vi "sequencerCWTopLevel.vi"() -> ()   [LabVIEW 2014]
uses:
  Controls/measVoltState.ctl
  sequencerState.ctl
  Controls/SPstate.ctl
  Controls/heinzingerSelect.ctl
  Controls/triggerTypes.ctl
  Controls/selectTrigger.ctl
  Controls/triggerEdge.ctl
  OutBits/OutbitsStateControl.ctl
  <vilib>/rvi/Emulation/niFpgaGetClockAttributes.vi
  <vilib>/rvi/Emulation/niFpgaSctlEmulationGetInTimedLoop.vi
  <vilib>/rvi/Emulation/niFpgaEmulationReportErrorSimple.vi
  Trigger/triggerGlobalVars.vi
  <vilib>/rvi/Emulation/niFpgaProcessEmulError.vi
  ScanTrigger/scanTriggerGlobalVars.vi
  StepTrigger/stepTriggerGlobalVars.vi
  sequencerGlobVars.vi
  MeasVolt/measVoltGlobVars.vi
  QueueHandler/queueHandlerGlobals.vi
  SimpleCounter/SCGlobVars.vi
  HeinzingerControl/heinzingerControlGlobals.vi
  OutBits/OutbitsGlobalVars.vi
  ScanDeviceLogic/scanDeviceGlobalVars.vi
  <vilib>/rvi/Emulation/niFpgaCriticalErrorInLSC.vi
panel:
  out "internalDacAvailable":bool
  in  "ScanDevice":enum16{"internal DAC", "external Python"}(ring)
  in  "scanDevSet":bool
  in  "scanDevTimeout(10ns)":i32
  in  "stepTrigDelay10ns":u32
  in  "softwareStepTrigger":bool
  in  "stepTriggerEdge":T1=enum."true-false"
  in  "stepTriggerTypes":T2
  in  "selectStepTrigger":T3
  in  "softwareScanTrigger":bool
  in  "scanTriggerEdge":T1=enum."true-false"
  in  "scanTrigDelay10ns":u32
  in  "selectScanTrigger":T3
  in  "scanTriggerTypes":T2
  out "nOfCmdsOutbit2":u32
  out "nOfCmdsOutbit1":u32
  out "nOfCmdsOutbit0":u32
  out "OutBitsState":T4
  in  "softwareTrigger":bool
  in  "pause":bool
  in  "stopVoltMeas":bool caption="measVoltStop"
  in  "measVoltCompleteDest":T5(ring)
  in  "dac0VRegister":u32=1572792 format="%024b"
  in  "triggerEdge":T1=enum."true-false"
  in  "trigDelay10ns":u32
  in  "selectTrigger":T3
  in  "triggerTypes":T2
  out "postAccOffsetVoltState":T6
  in  "postAccOffsetVoltControl":T6=enum."loading"
  out "SPerrorCount":u8
  out "SPstate":T7
  in  "dwellTime10ns":u32=2000000
  out "SPCtrQuWriteTimeout":bool
  in  "VoltOrScaler?":bool
  in  "dacStepSize20Bit":i32
  in  "dacStartRegister20Bit":i32
  in  "nOfSteps":i32
  in  "nOfScans":i32
  in  "invertScan":bool
  in  "waitForKepco(us)":u32
  in  "waitAfterReset(us)":u32 caption="waitForDmm(25nsTicks)"
  in  "measVoltPulseLength(25ns)":i32
  in  "measVoltTimeout(10ns)":i32 caption="measVoltTimeout(25ns)"
  in  "timedOutWhileHandshake":bool
  out "seqState":T8
  in  "cmdByHost":T8
  in  "abort":bool
  in  "halt":bool
  in  "hostConfirmsHzOffsetIsSet":bool
  out "measVoltState":T9
  out "DACQuWriteTimeout":bool
  # "Step Trigger"
  # "Step Trigger"
  # "Scan Trigger"
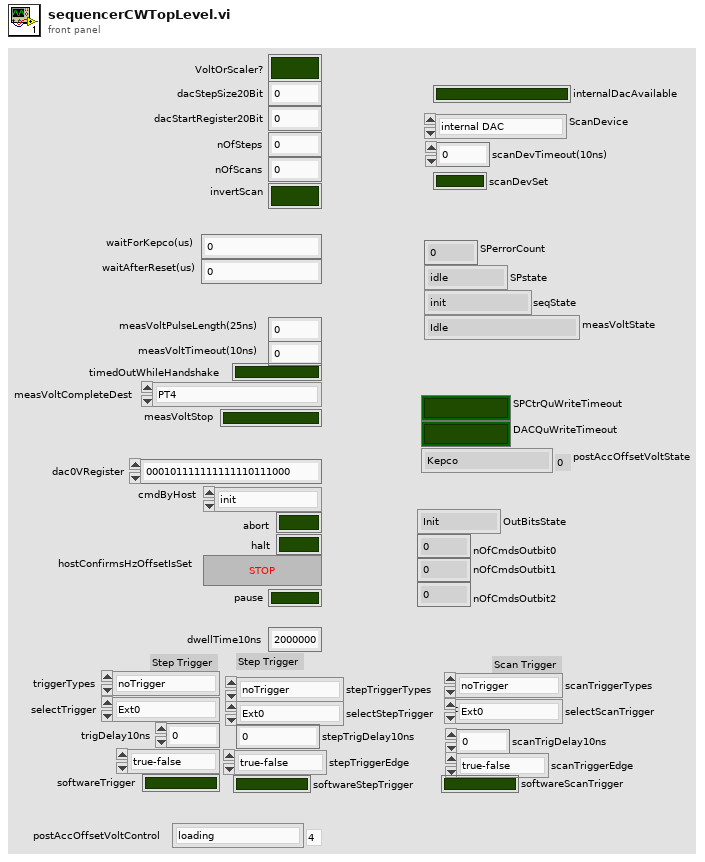
[diagram p1: front panel]
types:
  T1 = typedef "triggerEdge.ctl" = enum8{"either", "false-true", "true-false"}
  T2 = typedef "triggerTypes.ctl" = enum16{"noTrigger", "singleHitDelay", "singleHit", "software", "sweep"}
  T3 = typedef "selectTrigger.ctl" = enum8{"Ext0", "Ext1", "Ext2", "Ext3", "Ext4", "Ext5", "Ext6", "Ext7", "Int0", "Int1", "Int2", "Int3", "Int4", "Int5", "Int6", "Int7"}
  T4 = typedef "OutbitsStateControl.ctl" = enum16{"Init", "Idle", "loading", "listening", "clearing", "error"}
  T5 = enum16{"PT4", "C1D30", "C1D31", "PT4_C1D30", "PT4_C1D31", "PT4_C1D30_C1D31", "C1D30_C1D31"}
  T6 = typedef "heinzingerSelect.ctl" = enum8{"Kepco", "Heinzinger0", "Heinzinger1", "Heinzinger2", "loading"}
  T7 = typedef "SPstate.ctl" = enum16{"idle", "scanning", "done", "error"}
  T8 = typedef "sequencerState.ctl" = enum16{"init", "idle", "measureOffset", "measureTrack", "measComplete", "error"}
  T9 = typedef "measVoltState.ctl" = enum16{"Idle", "sendMeasRequest", "waitUntilDone", "done"}
  T10 = cluster{"SCLK":refnum<k21>, "CS":refnum<k21>, "MOSI":refnum<k21>, "MISO":refnum<k21>}
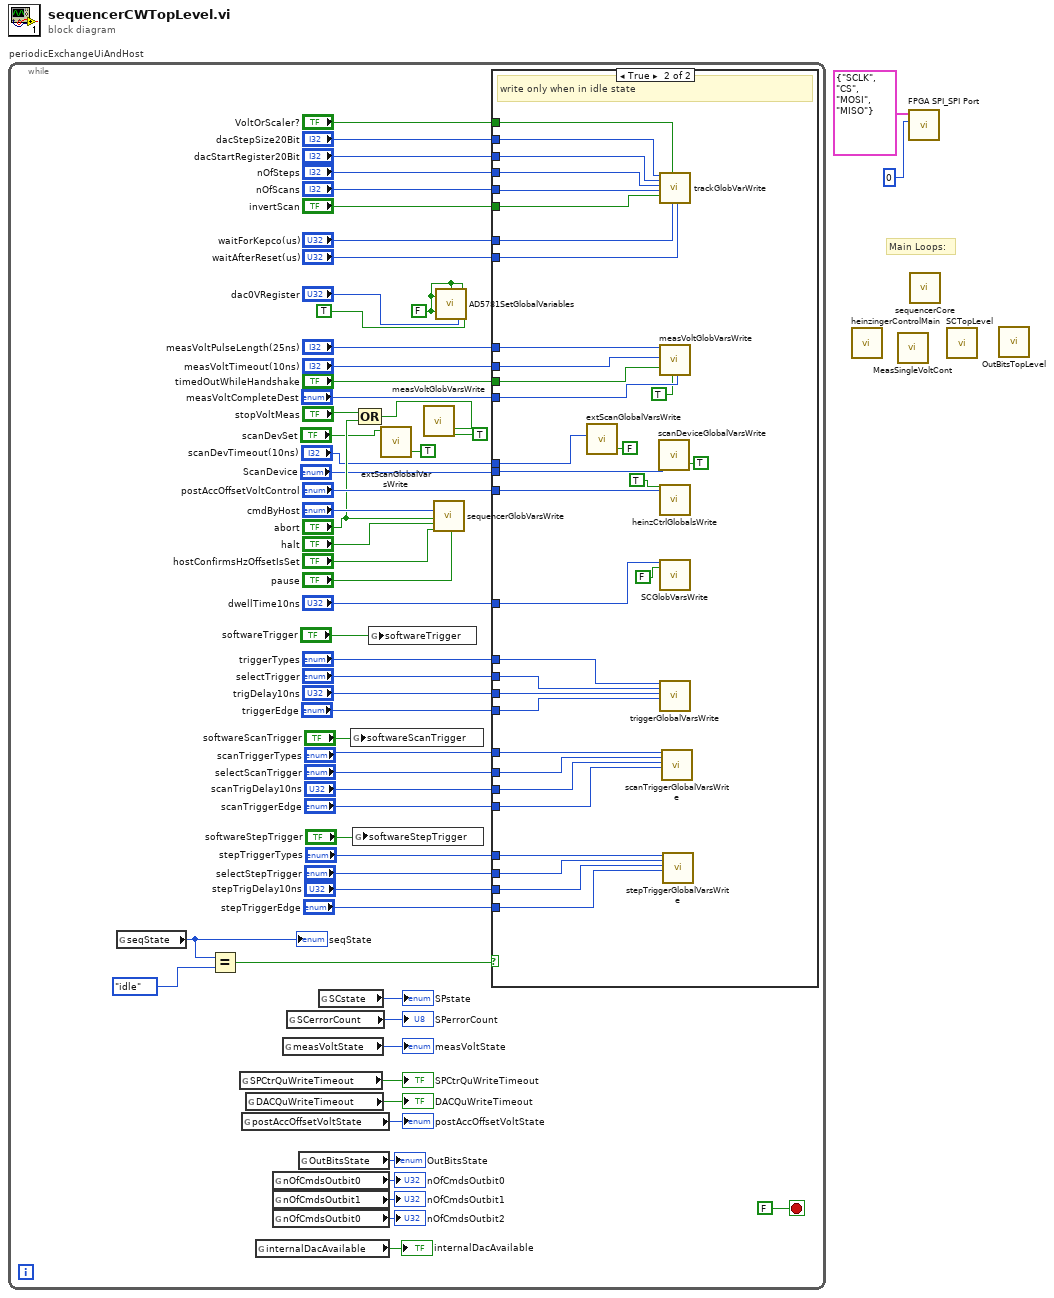
[diagram p0: block diagram]
diagram:
  # "Main Loops:"
  n1 = while "periodicExchangeUiAndHost" {
    stop <- FALSE stop-if-true
    w31 = FALSE ("write setDACRegister")
    n2 = global read "sequencerGlobVars.vi" "seqState"() -> (w43:T8)
    "seqState" <- w43
    n3 = Equal?(x=w43, y=sequencerState."idle") -> (x = y?=w60:bool)
    n4 = global read "queueHandlerGlobals.vi" "SPCtrQuWriteTimeout"() -> (→"SPCtrQuWriteTimeout":bool)
    n5 = global read "heinzingerControlGlobals.vi" "postAccOffsetVoltState"() -> (→"postAccOffsetVoltState":T6)
    n6 = global read "queueHandlerGlobals.vi" "DACQuWriteTimeout"() -> (→"DACQuWriteTimeout":bool)
    n7 = global read "scanDeviceGlobalVars.vi" "internalDacAvailable"() -> (→"internalDacAvailable":bool)
    n8 = global read "OutbitsGlobalVars.vi" "nOfCmdsOutbit0"() -> (→"nOfCmdsOutbit0":u32)
    n9 = global read "OutbitsGlobalVars.vi" "nOfCmdsOutbit1"() -> (→"nOfCmdsOutbit1":u32)
    n10 = global read "OutbitsGlobalVars.vi" "nOfCmdsOutbit0"() -> (→"nOfCmdsOutbit2":u32)
    n11 = global read "measVoltGlobVars.vi" "measVoltState"() -> (→"measVoltState":T9)
    n12 = global read "SCGlobVars.vi" "SCerrorCount"() -> (→"SPerrorCount":u8)
    n13 = global read "OutbitsGlobalVars.vi" "OutBitsState"() -> (→"OutBitsState":T4)
    n14 = global read "SCGlobVars.vi" "SCstate"() -> (→"SPstate":T7)
    n15 = global write "scanTriggerGlobalVars.vi" "softwareScanTrigger"("softwareScanTrigger") -> ()
    n16 = global write "stepTriggerGlobalVars.vi" "softwareStepTrigger"("softwareStepTrigger") -> ()
    n17 = Compound Arithmetic op=OR("stopVoltMeas", "abort") -> (w25:bool)
    n18 = global write "triggerGlobalVars.vi" "softwareTrigger"("softwareTrigger") -> ()
    n19 = call "extScanGlobalVarsWrite.vi"("WriteDevSet"=TRUE, "scanDevSet"="scanDevSet") -> ()  [unwired: 10 in]
    n20 = call "measVoltGlobVarsWrite.vi"("stopVoltMeas"=w25, "writeStopVoltMeas"=TRUE) -> ()  [unwired: 18 in]
    n21 = call "sequencerGlobVarsWrite.vi"("cmdByHost"="cmdByHost", "abort"="abort", "halt"="halt", "hostConfirmsHzOffsetIsSet"="hostConfirmsHzOffsetIsSet", "pause"="pause") -> ()  [unwired: 15 in]
    n22 = call "AD5781SetGlobalVariables.vi"("write actDACRegister"=w31, "write setDACRegister"=w31, "write DacStateCmdByHost"=w31, "dac0VRegister"="dac0VRegister", "writeSpiGlobals"=w31, "write dac0VRegister"=TRUE) -> ()  [unwired: 14 in]
    n23 = case shown="True" w60 {
      tunnel: "VoltOrScaler?" -> [_ w94]
      tunnel: "dacStepSize20Bit" -> [_ w93]
      tunnel: "dacStartRegister20Bit" -> [_ w92]
      tunnel: "nOfSteps" -> [_ w91]
      tunnel: "nOfScans" -> [_ w90]
      tunnel: "invertScan" -> [_ w89]
      tunnel: "waitForKepco(us)" -> [_ w88]
      tunnel: "waitAfterReset(us)" -> [_ w87]
      tunnel: "measVoltPulseLength(25ns)" -> [_ w86]
      tunnel: "measVoltTimeout(10ns)" -> [_ w85]
      tunnel: "timedOutWhileHandshake" -> [_ w84]
      tunnel: "dwellTime10ns" -> [_ w82]
      tunnel: "postAccOffsetVoltControl" -> [_ w80]
      tunnel: "triggerTypes" -> [_ w79]
      tunnel: "selectTrigger" -> [_ w78]
      tunnel: "trigDelay10ns" -> [_ w77]
      tunnel: "triggerEdge" -> [_ w76]
      tunnel: "measVoltCompleteDest" -> [_ w75]
      tunnel: "scanTriggerTypes" -> [_ w73]
      tunnel: "selectScanTrigger" -> [_ w72]
      tunnel: "scanTrigDelay10ns" -> [_ w71]
      tunnel: "scanTriggerEdge" -> [_ w70]
      tunnel: "stepTriggerTypes" -> [_ w69]
      tunnel: "selectStepTrigger" -> [_ w68]
      tunnel: "stepTrigDelay10ns" -> [_ w67]
      tunnel: "stepTriggerEdge" -> [_ w66]
      tunnel: "ScanDevice" -> [_ w65]
      tunnel: "scanDevTimeout(10ns)" -> [_ w64]
      frame False {
      }
      frame True {
        # "write only when in idle state"
        n24 = call "extScanGlobalVarsWrite.vi"("WriteDevSet"=FALSE, "scanDevTimeout(10ns)"=w64) -> ()  [unwired: 10 in]
        n25 = call "scanDeviceGlobalVarsWrite.vi"("ChooseScanDevice"=TRUE, "ScanDevice"=w65) -> ()  [unwired: 10 in]
        n26 = call "trackGlobVarWrite.vi"("dacStepSize20Bit"=w93, "dacStartRegister20Bit"=w92, "nOfSteps"=w91, "nOfScans"=w90, "invertScan"=w89, "VoltOrScaler?"=w94, "waitForKepco(us)"=w88, "waitAfterReset(us)"=w87) -> ()  [unwired: 12 in]
        n27 = call "measVoltGlobVarsWrite.vi"("measVoltPulseLength(25ns)"=w86, "measVoltTimeout(10ns)"=w85, "timedOutWhileHandshake"=w84, "writeMeasVoltCompleteDest"=TRUE, "measVoltCompleteDest"=w75) -> ()  [unwired: 15 in]
        n28 = call "heinzCtrlGlobalsWrite.vi"("w_postAccOffsetVoltControl"=TRUE, "postAccOffsetVoltControl"=w80) -> ()  [unwired: 26 in]
        n29 = call "SCGlobVarsWrite.vi"("dwellTime10ns"=w82, "stop"=FALSE) -> ()  [unwired: 18 in]
        n30 = call "triggerGlobalVarsWrite.vi"("triggerTypes"=w79, "selectTrigger"=w78, "delay_10ns_ticks"=w77, "triggerEdge"=w76) -> ()  [unwired: 16 in]
        n31 = call "scanTriggerGlobalVarsWrite.vi"("scanTriggerTypes"=w73, "selectScanTrigger"=w72, "scan_trig_delay_10ns_ticks"=w71, "scanTriggerEdge"=w70) -> ()  [unwired: 16 in]
        n32 = call "stepTriggerGlobalVarsWrite.vi"("stepTriggerTypes"=w69, "selectStepTrigger"=w68, "step_trig_delay_10ns_ticks"=w67, "stepTriggerEdge"=w66) -> ()  [unwired: 16 in]
      }
    }
  }
  n33 = call "heinzingerControlMain.vi"() -> ()  [unwired: 3 in]
  n34 = call "MeasSingleVoltCont.vi"() -> ()  [unwired: 12 in]
  n35 = call "FPGA SPI_SPI Port.vi"("Port"=i8 0, "FPGA IO"=T10 {"SCLK"="SCLK", "CS"="CS", "MOSI"="MOSI", "MISO"="MISO"}) -> ()  [unwired: 10 in]
  n36 = call "sequencerCore.vi"() -> ()  [unwired: 12 in]
  n37 = call "SCTopLevel.vi"() -> ()  [unwired: 12 in]
  n38 = call "OutBitsTopLevel.vi"() -> ()  [unwired: 12 in]
